vi "BenjaminR - LabVIEW Menus (Help).vi"   [LabVIEW 2017]
doc: "https://bit.ly/3Px2ylV"
uses:
  vi.lib/addons/BenjaminR/shared/shared.lvlib
  vi.lib/addons/BenjaminR/vi_tools/vi_tools.lvlib
types:
  T1 = cluster{"VI Description":string, "VI Help.Tag":string, "VI Help.Doc":string}
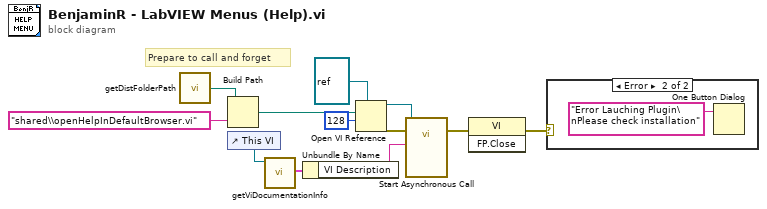
[diagram p0: block diagram]
diagram:
  # "Prepare to call and forget"
  n1 = call "getDistFolderPath.vi"() -> ("Dist Folder Path"=w4:path)
  n2 = Build Path(base path=w4, name or relative path="shared\\openHelpInDefaultBrowser.vi") -> (appended path=w7:path)
  n3 = control-ref of="This VI"() -> (w3:refnum<vi>)
  n4 = call "getViDocumentationInfo.vi"("VI in"=w3) -> ("VI Documentation Info"=w2:T1)  [unwired: 7 in, 3 out]
  n5 = Unbundle By Name(w2) -> ("VI Description"=w1:string)
  n6 = Open VI Reference(type specifier VI Refnum (for type only)=refnum<vi> refnum ("VI Refnum"), vi path=w7, options=128) -> (vi reference=w11:refnum<vi>, error out=w9:errorcluster)  [unwired: 3 in]
  n7 = call-by-ref "Start Asynchronous Call"(reference=w11, error in=w9, "name or relative path"=w1) -> (error out=w8:errorcluster)  [unwired: 10 in, 2 out]
  n8 = invoke class="VI" method="FP.Close"(error in=w8) -> (error out=w5:errorcluster)  [unwired: 2 in, 2 out]
  n9 = case shown="Error" w5 {
    frame No Error {
    }
    frame Error {
      n10 = One Button Dialog(message="Error Lauching Plugin\nPlease check installation") -> ()  [unwired: 1 in, 1 out]
    }
  }
